vi "moveY.vi"(8 "error in (no error)":errorcluster, 11 "Y":dbl) -> (0 "error out":errorcluster)   [LabVIEW 2019]
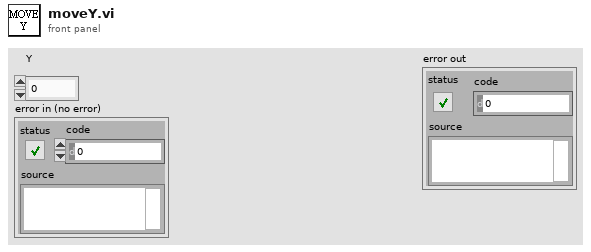
[diagram p1: front panel]
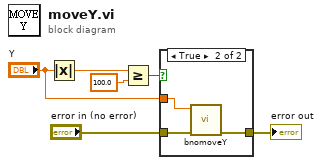
[diagram p0: block diagram]
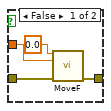
[diagram p2: hidden frame]
diagram:
  n1 = Absolute Value(x="Y") -> (abs(x)=w2:dbl)
  n2 = Greater Or Equal?(x=w2, y=100.0) -> (x >= y?=w6:bool)
  n3 = case shown="True" w6 {
    tunnel: "Y" -> [w10 w13]
    tunnel: "error in (no error)" -> [w8 w11]
    tunnel: [w7 w12] -> w3
    frame False {
      n4 = call "MoveF.vi"("X"=0.0, "Y"=w10, "error in (no error)"=w8) -> ("error out"=w7:errorcluster)  [unwired: 12 in]
    }
    frame True {
      n5 = call "bnomoveY.vi"("error in (no error)"=w11, "Y"=w13) -> ("error out"=w12:errorcluster)  [unwired: 9 in]
    }
  }
  "error out" <- w3
